vi "Pulse Train Generation TIO.vi"(6 "Delay":u32=200, 8 "error in":errorcluster) -> (0 "error out":errorcluster, 3 "Pulse Generation Task ID's Out":u32[](array[numeric]) format="%.0x")   [LabVIEW 2009]
uses:
  Acquisition Settings.vi
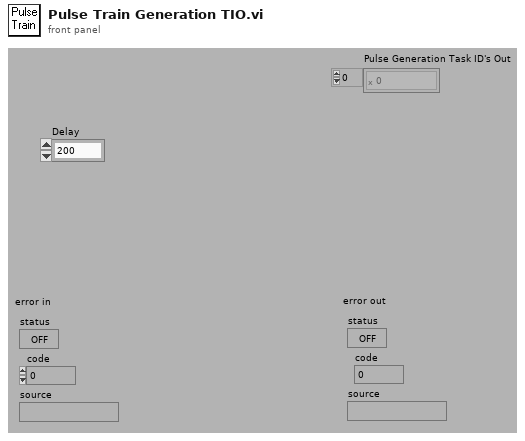
[diagram p1: front panel]
types:
  T1 = cluster{"Name":string, "Device Number":i16, "Counter Number":i16, "Pulse Spec 1 (Clocks)":u32, "Pulse Spec 2 (Clocks)":u32, "Signal Routing Configuration":i16, "Inverted":bool}[]
  T2 = cluster{"Name":string, "Signal Routing":cluster{"signal name":u16, "signal source":u16, "signal source line number":u32, "signal name line number":u32}[]}[]
  T3 = cluster{"Name":string, "Signal Routing":cluster{"signal name":u16, "signal source":u16, "signal source line number":u32, "signal name line number":u32}[]}
  T4 = cluster{"signal name":u16, "signal source":u16, "signal source line number":u32, "signal name line number":u32}[]
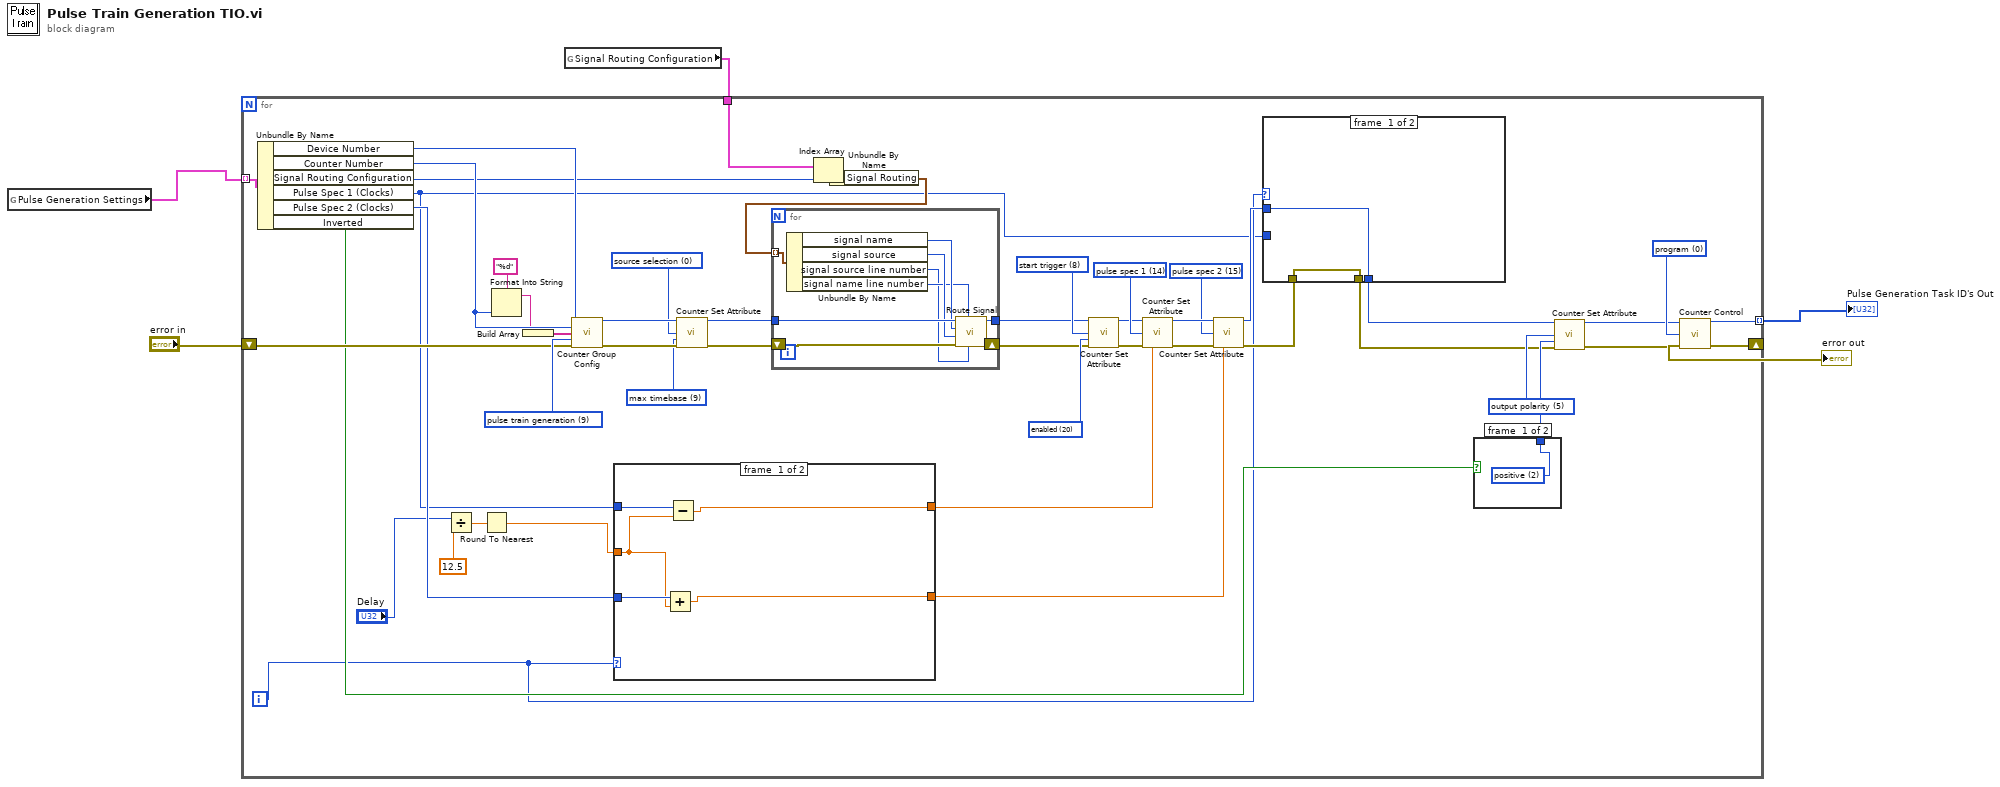
[diagram p0: block diagram]
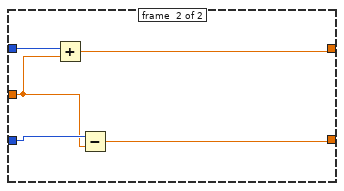
[diagram p2: hidden frame]
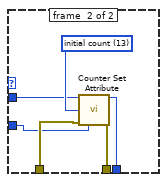
[diagram p3: hidden frame]
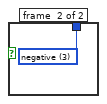
[diagram p4: hidden frame]
diagram:
  n1 = global read "Acquisition Settings.vi" "Pulse Generation Settings"() -> (w2:T1)
  n2 = global read "Acquisition Settings.vi" "Signal Routing Configuration"() -> (w1:T2)
  n3 = for {
    tunnel: w2 -> [w52] mode=indexing
    tunnel: [w51] -> w3 mode=indexing
    shift-right: [w32] -> w4
    shift-left: "error in" -> [w33]
    tunnel: w1 -> [w24]
    i -> [w14]
    w21 = u32 5 items=["source selection", "source polarity", "gate selection", "gate polarity", "output mode", "output polarity", "aux line selection", "aux line polarity", "start trigger", "counting synchronous", "up down", "buffer mode", "encoder type", "initial count", "pulse spec 1", "pulse spec 2", "pulse spec 3", "pulse spec 4", "auto increment", "prescale value", "Z index active", "Z index value", "Z index reload phase", "synchronization line", "synchronization method", "initial seconds", "precision", "transfer method", "start trigger polarity", "timeout", "initial seconds enable"] ("attribute ID")
    w34 = u32 20 items=["yes", "no", "positive", "negative", "high", "low", "low to high", "high to low", "default", "max timebase", "other counter gate", "other counter TC", "other counter output", "other counter source", "source", "gate", "aux line", "in start trigger", "in stop trigger", "automatic", "enabled", "count up", "count down", "hardware", "single", "continuous", "pulse", "toggle", "quadrature encoder X1", "quadrature encoder X2", "quadrature encoder X4", "two pulse counting", "A high B high", "A high B low", "A low B high", "A low B low", "PFI n", "RTSI n", "timebase n", "disabled", "PXI backplane clock", "counter n output", "(Reserved) pulse per second", "(Reserved) IRIG-B", "(Reserved) seconds", "(Reserved) nano seconds", "interrupts", "dma", "RTSI clock"] ("attribute value type")
    w35 = u32 8 items=["source selection", "source polarity", "gate selection", "gate polarity", "output mode", "output polarity", "aux line selection", "aux line polarity", "start trigger", "counting synchronous", "up down", "buffer mode", "encoder type", "initial count", "pulse spec 1", "pulse spec 2", "pulse spec 3", "pulse spec 4", "auto increment", "prescale value", "Z index active", "Z index value", "Z index reload phase", "(Reserved) synchronization line", "(Reserved) synchronization method", "(Reserved) seconds", "(Reserved) precision", "transfer method", "start trigger polarity"] ("attribute ID")
    w38 = u32 9 items=["simple event counting", "single period measurement", "single pulse width measurement", "triggered pulse width measurement", "two signal edge separation measurement", "position measurement", "single pulse generation", "single triggered pulse generation", "retriggerable pulse generation", "pulse train generation", "frequency shift keying", "buffered event counting", "buffered period measurement", "buffered semiperiod measurement", "buffered pulse width measurement", "buffered two signal edge separation measurement", "buffered position measurement"] ("task type")
    w42 = u32 15 items=["source selection", "source polarity", "gate selection", "gate polarity", "output mode", "output polarity", "aux line selection", "aux line polarity", "start trigger", "counting synchronous", "up down", "buffer mode", "encoder type", "initial count", "pulse spec 1", "pulse spec 2", "pulse spec 3", "pulse spec 4", "auto increment", "prescale value", "Z index active", "Z index value"] ("attribute ID")
    w43 = u32 14 items=["source selection", "source polarity", "gate selection", "gate polarity", "output mode", "output polarity", "aux line selection", "aux line polarity", "start trigger", "counting synchronous", "up down", "buffer mode", "encoder type", "initial count", "pulse spec 1", "pulse spec 2", "pulse spec 3", "pulse spec 4", "auto increment", "prescale value", "Z index active", "Z index value"] ("attribute ID")
    w44 = u32 9 items=["yes", "no", "positive", "negative", "high", "low", "low to high", "high to low", "default", "max timebase", "other counter gate", "other counter TC", "other counter output", "other counter source", "source", "gate", "aux line", "in start trigger", "in stop trigger", "automatic", "enabled", "count up", "count down", "hardware", "single", "double", "pulse", "toggle", "quadrature encoder X1", "quadrature encoder X2", "quadrature encoder X4", "two pulse counting", "A high B high", "A high B low", "A low B high", "A low B low", "PFI n", "RTSI n", "timebase n"] ("attribute value type")
    w45 = u32 0 items=["source selection", "source polarity", "gate selection", "gate polarity", "output mode", "output polarity", "aux line selection", "aux line polarity", "start trigger", "counting synchronous", "up down", "buffer mode", "encoder type", "initial count", "pulse spec 1", "pulse spec 2", "pulse spec 3", "pulse spec 4", "auto increment", "prescale value", "Z index active", "Z index value"] ("attribute ID")
    w54 = u32 0 items=["program", "reset", "arm", "prepare", "disarm", "count up", "count down", "switch cycle", "snapshot"] ("control code")
    n4 = Unbundle By Name(w52) -> ("Device Number"=w53:i16, "Counter Number"=w50:i16, "Signal Routing Configuration"=w25:i16, "Pulse Spec 1 (Clocks)"=w10:u32, "Pulse Spec 2 (Clocks)"=w13:u32, "Inverted"=w19:bool)
    n5 = Divide(x="Delay", y=12.5) -> (x/y=w8:dbl)
    n6 = Round To Nearest(number=w8) -> (nearest integer value=w6:dbl)
    n7 = Format Into String(format string="%d" ("Format String"), w50) -> (resulting string=w40:string)  [unwired: 2 in, 1 out]
    n8 = Build Array(w40) -> (w41:string[])
    n9 = call <vilib>:"Counter Group Config.vi"("device"=w53, "group"=w50, "counter list"=w41, "task type"=w38, "error in (no error)"=w33) -> ("task ID"=w49:u32, "error out"=w48:errorcluster)  [unwired: 8 in, 1 out]
    n10 = case shown="0, Default" w14 {
      tunnel: w10 -> [w59 w64]
      tunnel: w13 -> [w57 w63]
      tunnel: [w58 w62] -> w12
      tunnel: [w56 w61] -> w11
      tunnel: w6 -> [w55 w60]
      frame #0 {
        n11 = Add(x=w57, y=w55) -> (x+y=w56:dbl)
        n12 = Subtract(x=w59, y=w55) -> (x-y=w58:dbl)
      }
      frame #1 {
        n13 = Add(x=w64, y=w60) -> (x+y=w62:dbl)
        n14 = Subtract(x=w63, y=w60) -> (x-y=w61:dbl)
      }
    }
    n15 = call <vilib>:"Counter Set Attribute.vi"("task ID in"=w49, "attribute ID"=w45, "attribute value type"=w44, "error in (no error)"=w48) -> ("task ID out"=w29:u32, "error out"=w28:errorcluster)  [unwired: 10 in]
    n16 = Index Array(array=w24, index=w25) -> (element=w30:T3)
    n17 = Unbundle By Name(w30) -> ("Signal Routing"=w31:T4)
    n18 = for {
      tunnel: w29 -> [w83]
      shift-right: [w75] -> w26
      shift-left: w28 -> [w82]
      tunnel: w31 -> [w81] mode=indexing
      tunnel: [w76] -> w27
      n19 = Unbundle By Name(w81) -> ("signal name"=w80:u16, "signal source"=w79:u16, "signal source line number"=w77:u32, "signal name line number"=w78:u32)
      n20 = call <vilib>:"Route Signal.vi"("signal source line number"=w77, "signal name line number"=w78, "error in (no error)"=w82, "signal source"=w79, "signal name"=w80, "task ID"=w83) -> ("error out"=w75:errorcluster, "task ID out"=w76:u32)  [unwired: 4 in]
    }
    n21 = call <vilib>:"Counter Set Attribute.vi"("task ID in"=w27, "attribute ID"=w35, "attribute value type"=w34, "error in (no error)"=w26) -> ("task ID out"=w37:u32, "error out"=w36:errorcluster)  [unwired: 10 in]
    n22 = call <vilib>:"Counter Set Attribute.vi"("task ID in"=w37, "attribute ID"=w43, "error in (no error)"=w36, "attribute value number"=w12) -> ("task ID out"=w47:u32, "error out"=w46:errorcluster)  [unwired: 10 in]
    n23 = call <vilib>:"Counter Set Attribute.vi"("task ID in"=w47, "attribute ID"=w42, "error in (no error)"=w46, "attribute value number"=w11) -> ("task ID out"=w18:u32, "error out"=w16:errorcluster)  [unwired: 10 in]
    n24 = case shown="1" w14 {
      tunnel: w18 -> [w66 w71]
      tunnel: [w66 w70] -> w17
      tunnel: w16 -> [w65 w69]
      tunnel: [w65 w68] -> w15
      tunnel: w10 -> [_ w67]
      frame #0 {
      }
      frame #1 {
        w72 = u32 13 items=["source selection", "source polarity", "gate selection", "gate polarity", "output mode", "output polarity", "aux line selection", "aux line polarity", "start trigger", "counting synchronous", "up down", "buffer mode", "encoder type", "initial count", "pulse spec 1", "pulse spec 2", "pulse spec 3", "pulse spec 4", "auto increment", "prescale value", "Z index active", "Z index value", "Z index reload phase", "synchronization line", "synchronization method", "initial seconds", "precision", "transfer method", "start trigger polarity", "timeout", "initial seconds enable"] ("attribute ID")
        n25 = call <vilib>:"Counter Set Attribute.vi"("task ID in"=w71, "attribute ID"=w72, "error in (no error)"=w69, "attribute value number"=w67) -> ("task ID out"=w70:u32, "error out"=w68:errorcluster)  [unwired: 10 in]
      }
    }
    n26 = case shown="False" w19 {
      tunnel: [w73 w74] -> w20
      frame #0 {
        w73 = u32 2 items=["yes", "no", "positive", "negative", "high", "low", "low to high", "high to low", "default", "max timebase", "other counter gate", "other counter TC", "other counter output", "other counter source", "source", "gate", "aux line", "in start trigger", "in stop trigger", "automatic", "enabled", "count up", "count down", "hardware", "single", "continuous", "pulse", "toggle", "quadrature encoder X1", "quadrature encoder X2", "quadrature encoder X4", "two pulse counting", "A high B high", "A high B low", "A low B high", "A low B low", "PFI n", "RTSI n", "timebase n", "disabled", "PXI backplane clock", "counter n output", "pulse per second", "IRIG-B", "seconds", "nanoseconds", "interrupts", "dma", "RTSI clock"] ("attribute value type")
      }
      frame #1 {
        w74 = u32 3 items=["yes", "no", "positive", "negative", "high", "low", "low to high", "high to low", "default", "max timebase", "other counter gate", "other counter TC", "other counter output", "other counter source", "source", "gate", "aux line", "in start trigger", "in stop trigger", "automatic", "enabled", "count up", "count down", "hardware", "single", "continuous", "pulse", "toggle", "quadrature encoder X1", "quadrature encoder X2", "quadrature encoder X4", "two pulse counting", "A high B high", "A high B low", "A low B high", "A low B low", "PFI n", "RTSI n", "timebase n", "disabled", "PXI backplane clock", "counter n output", "pulse per second", "IRIG-B", "seconds", "nanoseconds", "interrupts", "dma", "RTSI clock"] ("attribute value type")
      }
    }
    n27 = call <vilib>:"Counter Set Attribute.vi"("task ID in"=w17, "attribute ID"=w21, "attribute value type"=w20, "error in (no error)"=w15) -> ("task ID out"=w23:u32, "error out"=w22:errorcluster)  [unwired: 10 in]
    n28 = call <vilib>:"Counter Control.vi"("task ID"=w23, "control code"=w54, "error in (no error)"=w22) -> ("task ID out"=w51:u32, "error out"=w32:errorcluster)  [unwired: 11 in]
  }
  "error out" <- w4
  "Pulse Generation Task ID's Out" <- w3
